vi "Spectrograph_logEvent_disperserInPosition.vi"(8 "error in (no error)":errorcluster, 11 "logevent_disperserInPosition_Ctl":T1) -> (0 "error out":errorcluster, 2 "function return":i32, 3 "logevent_disperserInPosition_Ctl out":T1)   [LabVIEW 2016, in "SALLV_Spectrograph.lvlib"]
doc: "int Spectrograph_shm_logEvent_disperserInPositionLV(Spectrograph_logevent_disperserInPositionLV *logevent_disperserInPosition_Ctl );"
uses:
  SALLV_Spectrograph.lvlib
  DataTypes/logevent_disperserInPosition.ctl
  SALLV_Spectrograph.so
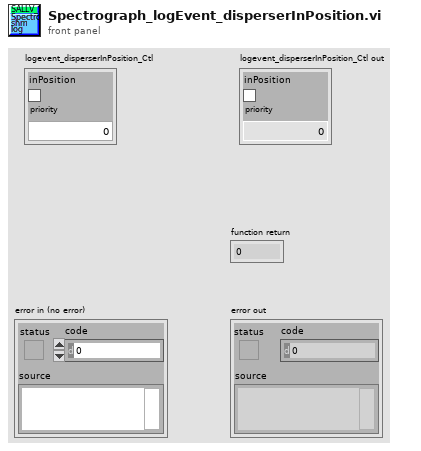
[diagram p1: front panel]
types:
  T1 = typedef "SALLV_Spectrograph.lvlib/logevent_disperserInPosition.ctl" = cluster{"inPosition":bool, "priority":i32}
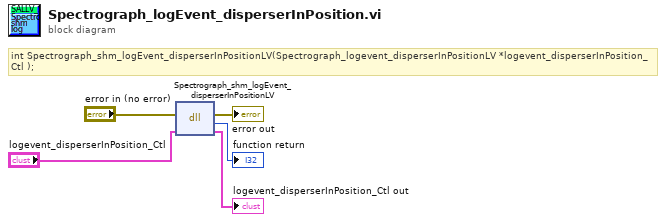
[diagram p0: block diagram]
diagram:
  # "int Spectrograph_shm_logEvent_disperserInPositionLV(Spectrograph_logevent_disperserInPositionLV *logevent_disperserInPosition_Ctl );"
  n1 = dll-call lib="home/harini/TCS/SALLV_Spectrograph/SALLV_Spectrograph.*" fn="Spectrograph_shm_logEvent_disperserInPositionLV"(error in="error in (no error)", "logevent_disperserInPosition_Ctl"="logevent_disperserInPosition_Ctl") -> (error out=→"error out":errorcluster, →"function return":i32, "logevent_disperserInPosition_Ctl"=→"logevent_disperserInPosition_Ctl out":T1)  [unwired: 2 in, 1 out]
